vi "Automatic Dummy Pick and Place.vi"() -> ()   [LabVIEW 2021]
uses:
  Classes/Assembly/Database Entry/Database Entry.lvclass
  Classes/Assembly/Assembly Run.lvclass
  <vilib>/Utility/file.llb/Read Delimited Spreadsheet (string).vi
  SubVIs/PUT_region.vi
  SubVIs/component_tray_region.vi
  SubVIs/assembly_tray_region.vi
  Classes/Controller/I-O/I-O.lvclass
  Classes/Controller/Controller.lvclass
panel:
  in  "Abort assembly":bool
  out "Status":string
  out "Stack names":T1
  out "Assembly Type":string
  out "Assembly tray region":dbl
  out "Component tray region":dbl
  out "PUT Region":dbl
  # "Click the Run arrow to start.\nFill out pop-up prompts.\nSee Status for more info.\nAnswer ALL prompts until program stops running!"
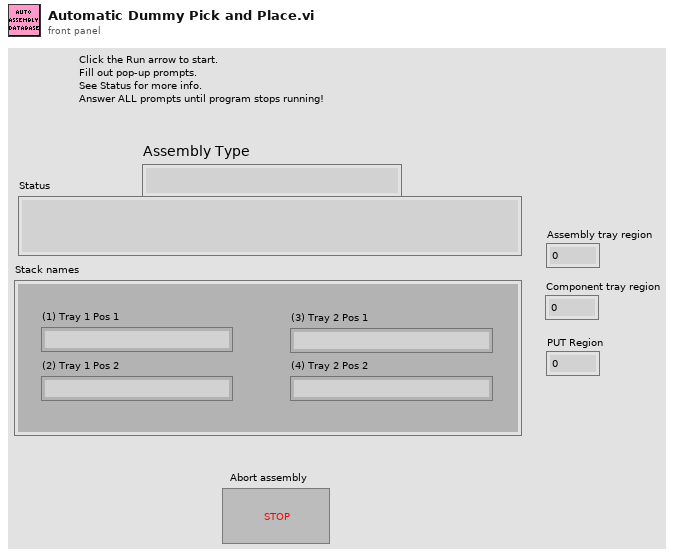
[diagram p1: front panel]
types:
  T1 = cluster{"(1) Tray 1 Pos 1":string, "(2) Tray 1 Pos 2":string, "(3) Tray 2 Pos 1":string, "(4) Tray 2 Pos 2":string}
  T2 = typedef "File Paths.ctl" = cluster{"Glue Pattern Folder":path, "Carrier Tray Folder":path, "Pick Up Tool Fixture Folder":path, "Components Folder":path, "Bellows Tool Offset.txt":path, "Pick Up Tool Offset.txt":path, "Dispense Tip Offset.txt":path, "Log Files":path, "Gantry Assembly Map.txt":path, "Syringe and offset map.txt":path, "Controllers Folder":path, "Local dbase config":path}
  T3 = typedef "Controller.lvclass/Controllers.ctl" = cluster{"I-O.lvclass":refnum<class "I-O.lvclass">, "Gantry":refnum<k24>, "Dispenser":refnum<visa-resource-name>}
  T4 = cluster{"Fixture ID":dbl, "Position":dbl, "Thickness":dbl}[]
  T5 = cluster{"Stack names[0]":string, "Stack names[1]":string, "Stack names[2]":string, "Stack names[3]":string}
  T6 = cluster{"Fixture ID":dbl, "Position":dbl, "Thickness":dbl}[][]
  T7 = cluster{"Fixture ID":dbl, "Position":dbl, "Thickness":dbl}
  T8 = typedef "I-O.lvclass/Pin Map.ctl" = cluster{"Region Valves":i32[], "Extra Valves":dbl[][][], "Tool Primary Valve":i32, "Tool Secondary Valve":i32, "Region Sensors":i32[], "Extra Sensors":dbl[][][], "Tool Primary Sensor":dbl, "Tool Secondary Sensor":dbl, "Compression Sensor":dbl, "5V":i32, "Dispenser Sensor":dbl, "Light Curtain":i32}
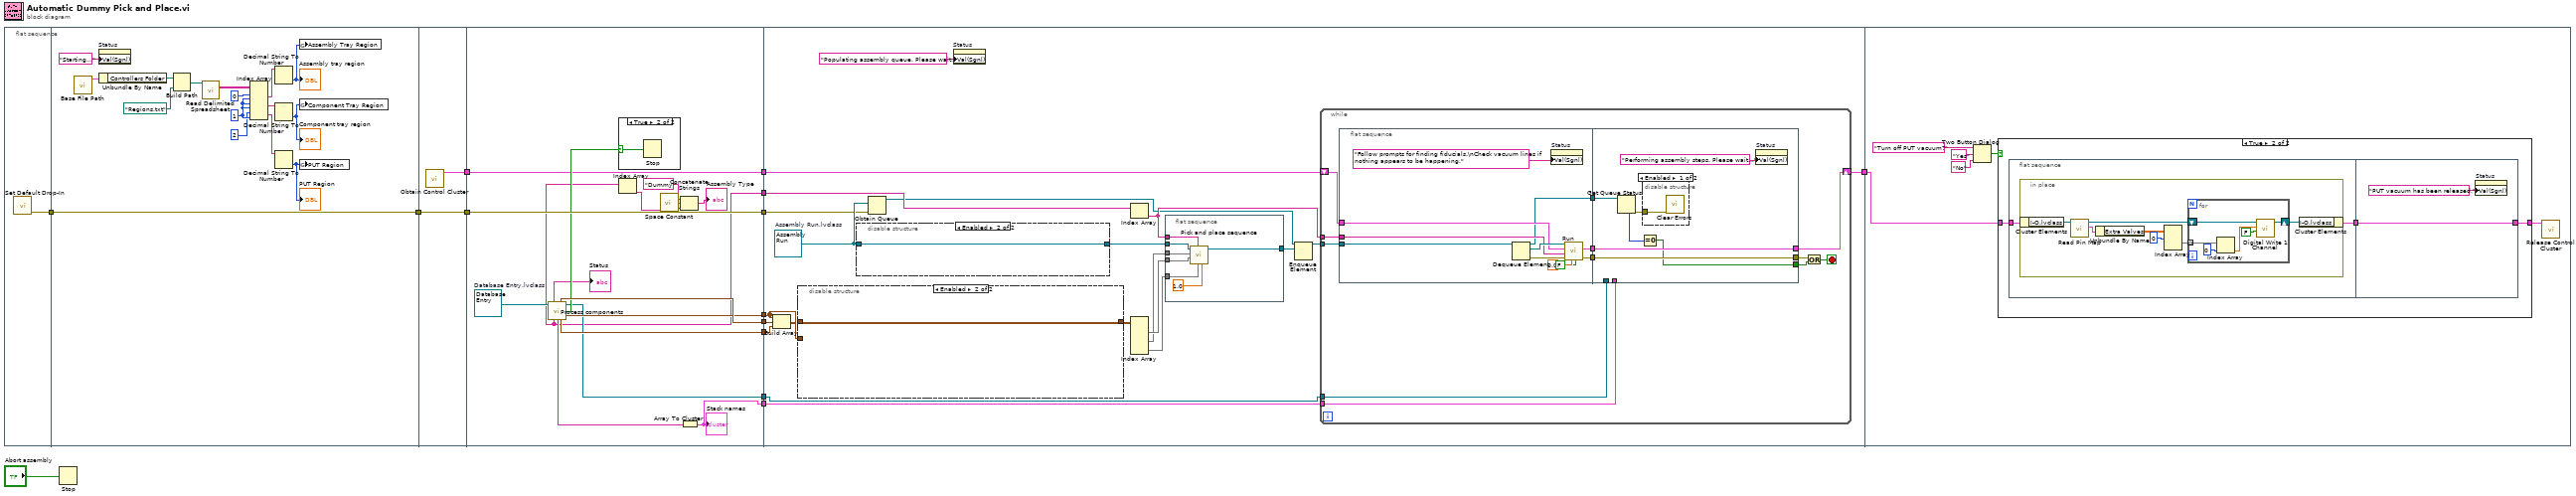
[diagram p0: block diagram]
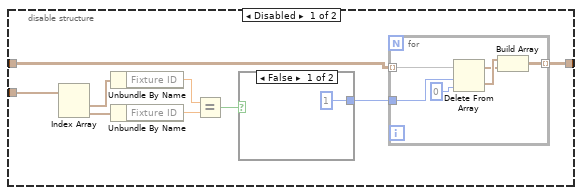
[diagram p3: hidden frame]
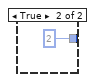
[diagram p4: hidden frame]
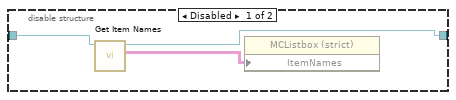
[diagram p5: hidden frame]
diagram:
  n1 = flat-sequence {
    tunnel: [w15] -> w13
    tunnel: [w17] -> w6
    tunnel: w13 -> [w17]
    tunnel: w6 -> [w33]
    tunnel: [w33] -> w5
    tunnel: [w32] -> w3
    tunnel: [w48] -> w14
    tunnel: w5 -> [w48]
    tunnel: [w47] -> w12
    tunnel: [w46] -> w11
    tunnel: [w45] -> w10
    tunnel: [w39] -> w9
    tunnel: [w42] -> w8
    tunnel: [w40] -> w7
    tunnel: [w34] -> w4
    tunnel: w3 -> [w34]
    tunnel: w14 -> [w70]
    tunnel: w12 -> [w69]
    tunnel: w11 -> [w68]
    tunnel: w10 -> [w64]
    tunnel: w9 -> [w67]
    tunnel: w8 -> [w61]
    tunnel: w7 -> [w62]
    tunnel: w4 -> [w63]
    tunnel: [w52] -> w1
    tunnel: w1 -> [w137]
    frame #0 {
      n2 = call "Set Default Drop-In.vi"() -> ("error out"=w15:errorcluster)  [unwired: 11 in]
    }
    frame #1 {
      w20 = 1 ("disabled index (col)")
      n3 = call "Base File Path.vi"() -> ("Paths Out"=w31:T2)  [unwired: 11 in]
      n4 = property on="Status" class="Str"("Val(Sgnl)"="Starting..." ("Value (Signaling)")) -> ()  [unwired: 2 in, 2 out]
      n5 = Unbundle By Name(w31) -> ("Controllers Folder"=w29:path)
      n6 = Build Path(base path=w29, name or relative path=path "Regions.txt") -> (appended path=w30:path)
      n7 = call-poly <vilib>:"Read Delimited Spreadsheet.vi"("file path (dialog if empty)"=w30) -> ("all rows"=w18:string[][])  [unwired: 9 in, 5 out]
      n8 = Index Array(array=w18, index (row) #1=0 ("index (row)"), index (col) #1=w20, index (row) #2=w20, index (col) #2=w20, index (row) #3=2 ("disabled index (row)"), index (col) #3=w20) -> (element #1=w23:string, element #2=w22:string, element #3=w24:string)
      n9 = Decimal String To Number(string=w23) -> (number=w26:i32)  [unwired: 2 in, 1 out]
      "Assembly tray region" <- w26
      n10 = Decimal String To Number(string=w22) -> (number=w27:i32)  [unwired: 2 in, 1 out]
      "Component tray region" <- w27
      n11 = Decimal String To Number(string=w24) -> (number=w25:i32)  [unwired: 2 in, 1 out]
      "PUT Region" <- w25
      n12 = global write "assembly_tray_region.vi" "Assembly Tray Region"(w26) -> ()
      n13 = global write "component_tray_region.vi" "Component Tray Region"(w27) -> ()
      n14 = global write "PUT_region.vi" "PUT Region"(w25) -> ()
    }
    frame #2 {
      n15 = call "Obtain Control Cluster.vi"() -> ("Control Out"=w32:T3)  [unwired: 10 in, 1 out]
    }
    frame #3 {
      w49 = refnum<class "Database Entry.lvclass"> refnum  # Database Entry.lvclass
      n16 = call "Process components.vi"("Database Entry in"=w49) -> ("Status"=→"Status":string, "PUT Settings"=w46:T4, "Database Entry out"=w40:refnum<class "Database Entry.lvclass">, "Aborted"=w43:bool, "Assembly Settings"=w45:T4, "Assembly Type"=w39:string[], "Stack names"=w44:string[], "Component Settings"=w47:T4)  [unwired: 4 in, 3 out]
      n17 = case shown="True" w43 {
        selector: w43 -> [_ w50]
        frame False {
        }
        frame True {
          n18 = Stop(stop? (T)=w50) -> ()
        }
      }
      n19 = Index Array(array=w39) -> (element=w38:string)  [unwired: 1 in]
      n20 = call <vilib>:"Space Constant.vi"() -> ("String"=w37:string)
      n21 = Concatenate Strings("Dummy", w37, w38) -> (→"Assembly Type":string)
      n22 = Array To Cluster(array=w44) -> (cluster=w42:T5)
      "Stack names" <- w42
    }
    frame #4 {
      w71 = refnum<class "Assembly Run.lvclass"> refnum  # Assembly Run.lvclass
      n23 = Build Array(w64, w68, w69) -> (w58:T6)
      n24 = disable-structure shown="Enabled" {
        disable-tunnel: w64 -> [w87 _]
        disable-tunnel: [w86 w96] -> w59
        disable-tunnel: w58 -> [w85 w96]
        frame Disabled {
          n25 = Index Array(array=w87) -> (element #1=w84:T7, element #2=w83:T7)  [unwired: 2 in]
          n26 = Unbundle By Name(w84) -> ("Fixture ID"=w82:dbl)
          n27 = Unbundle By Name(w83) -> ("Fixture ID"=w81:dbl)
          n28 = Equal?(x=w82, y=w81) -> (x = y?=w80:bool)
          n29 = case shown="False" w80 {
            tunnel: [1 2] -> w79
            frame False {
            }
            frame True {
            }
          }
          n30 = for {
            tunnel: w85 -> [w95] mode=indexing
            tunnel: [w94] -> w86 mode=indexing
            tunnel: w79 -> [w90]
            n31 = Delete From Array(array=w95, length=w90, index=0) -> (deleted portion=w92:T4, array with subset deleted=w91:T4)
            n32 = Build Array(w92, w91) -> (w94:T6)
          }
        }
        frame Enabled {
        }
      }
      n33 = disable-structure shown="Enabled" {
        disable-tunnel: w71 -> [w99 w100]
        disable-tunnel: [w97 w100] -> w60
        frame Disabled {
          n34 = call "Get Item Names.vi"("Assembly Run in"=w99) -> ("Item names"=w98:string[][], "Assembly Run out"=w97:refnum<class "Assembly Run.lvclass">)  [unwired: 8 in, 1 out]
          n35 = property class="MCListbox (strict)"("ItemNames"=w98) -> ()  [unwired: 2 in, 2 out]
        }
        frame Enabled {
        }
      }
      n36 = Obtain Queue(element data type=w71, error in (no error)=w70) -> (queue out=w65:refnum<queue>)  [unwired: 3 in, 2 out]
      n37 = property on="Status" class="Str"("Val(Sgnl)"="Populating assembly queue. Please wait." ("Value (Signaling)")) -> ()  [unwired: 2 in, 2 out]
      n38 = Index Array(array=w67) -> (element=w66:string)  [unwired: 1 in]
      n39 = Index Array(array=w59) -> (element #1=w57:T4, element #2=w56:T4, element #3=w55:T4)  [unwired: 6 in]
      n40 = flat-sequence {
        tunnel: [w77] -> w54
        tunnel: w66 -> [w76]
        tunnel: w56 -> [w73]
        tunnel: w55 -> [w72]
        tunnel: w60 -> [w78]
        tunnel: w57 -> [w74]
        frame #0 {
          n41 = call "Pick and place sequence.vi"("Numeric"=1.0, "Component Tray map"=w72, "Assembly Type"=w76, "Assembly Tray map"=w74, "PUT map"=w73, "Assembly Run in"=w78) -> ("Assembly Run out"=w77:refnum<class "Assembly Run.lvclass">)  [unwired: 4 in, 1 out]
        }
      }
      n42 = Enqueue Element(queue=w65, element=w54) -> (queue out=w53:refnum<queue>)  [unwired: 2 in, 2 out]
      n43 = while {
        shift-right: [w111] -> w52
        shift-left: w63 -> [w112]
        tunnel: w66 -> [w110]
        tunnel: w53 -> [w109]
        tunnel: w62 -> [w103]
        tunnel: w61 -> [w102]
        stop <- w104 stop-if-true
        n44 = flat-sequence {
          tunnel: w112 -> [w121]
          tunnel: w110 -> [w119]
          tunnel: w109 -> [w116]
          tunnel: [w120] -> w108
          tunnel: [w118] -> w107
          tunnel: [w117] -> w106
          tunnel: [w129] -> w105
          tunnel: [w130] -> w111
          tunnel: w108 -> [w130]
          tunnel: w107 -> [w129]
          tunnel: w106 -> [w128]
          tunnel: w103 -> [_]
          tunnel: w102 -> [_]
          tunnel: [w125] -> w101
          frame #0 {
            n45 = Dequeue Element(queue=w116) -> (queue out=w117:refnum<queue>, element=w123:refnum<class "Assembly Run.lvclass">, error out=w122:errorcluster)  [unwired: 2 in, 1 out]
            n46 = property on="Status" class="Str"("Val(Sgnl)"="Follow prompts for finding fiducials.\nCheck vacuum lines if nothing appears to be happening." ("Value (Signaling)")) -> ()  [unwired: 2 in, 2 out]
            n47 = call-dynamic "Run.vi"("Dispense?"=FALSE, "Pickup_Test_Number"=0.0, "error in (no error)"=w122, "Assembly Type"=w119, "Control In"=w121, "Assembly In"=w123) -> ("error out"=w118:errorcluster, "Control Out"=w120:T3)  [unwired: 3 in, 1 out]
          }
          frame #1 {
            n48 = Get Queue Status(queue=w128) -> (error out=w126:errorcluster, # elements in queue=w127:i32)  [unwired: 2 in, 6 out]
            n49 = Equal To 0?(x=w127) -> (x = 0?=w125:bool)
            n50 = disable-structure shown="Enabled" {
              disable-tunnel: w126 -> [w131 _]
              frame Enabled {
                n51 = call <vilib>:"Clear Errors.vi"("error in (no error)"=w131) -> ()  [unwired: 5 in, 2 out]
              }
              frame Disabled {
              }
            }
            n52 = property on="Status" class="Str"("Val(Sgnl)"="Performing assembly steps. Please wait...") -> ()  [unwired: 2 in, 2 out]
          }
        }
        n53 = Or(x=w105, y=w101) -> (x .or. y?=w104:bool)
      }
    }
    frame #5 {
      n54 = Two Button Dialog(message="Turn off PUT vacuum?", 1:"No" ("F button name (\"Cancel\")"), 2:"Yes" ("T button name (\"OK\")")) -> (T button?=w132:bool)
      n55 = case shown="True" w132 {
        tunnel: w137 -> [w138 w140]
        tunnel: [w138 w139] -> w136
        frame False {
        }
        frame True {
          n56 = flat-sequence {
            tunnel: w140 -> [w143]
            tunnel: [w142] -> w141
            tunnel: w141 -> [w158]
            tunnel: [w158] -> w139
            frame #0 {
              n57 = in-place {
                n58 = in-place-cluster #1(w143) -> ("I-O.lvclass"=w145:refnum<class "I-O.lvclass">)
                n59 = call-dynamic "Read Pin Map.vi"("I-O in"=w145) -> ("Pin Map 2"=w150:T8, "I-O out"=w147:refnum<class "I-O.lvclass">)  [unwired: 8 in, 1 out]
                n60 = Unbundle By Name(w150) -> ("Extra Valves"=w149:dbl[][][])
                n61 = Index Array(array=w149, index (dim 0)=0 ("index (page)")) -> (element=w148:dbl[][])  [unwired: 2 in]
                n62 = for {
                  tunnel: w148 -> [w156] mode=indexing
                  shift-right: [w154] -> w144
                  shift-left: w147 -> [w155]
                  n63 = Index Array(array=w156, index=0) -> (element=w153:dbl)
                  n64 = call-dynamic "Digital Write 1 Channel.vi"("Value"=FALSE, "Channel"=w153, "I-O.lvclass"=w155) -> ("I-O.lvclass 2"=w154:refnum<class "I-O.lvclass">)  [unwired: 7 in, 1 out]
                }
                n65 = in-place-cluster #1("I-O.lvclass"=w144) -> (w142:T3)
              }
            }
            frame #1 {
              n66 = property on="Status" class="Str"("Val(Sgnl)"="PUT vacuum has been released." ("Value (Signaling)")) -> ()  [unwired: 2 in, 2 out]
            }
          }
        }
      }
      n67 = call "Release Control Cluster.vi"("output cluster"=w136) -> ()  [unwired: 11 in]
    }
  }
  n68 = Stop(stop? (T)="Abort assembly") -> ()
